vi "Copy of Create calibration array.vi"() -> ()   [LabVIEW 2009, in "Varian Magnet.lvclass"]
uses:
  Varian Magnet.lvclass
panel:
  in  "# of points":dbl
  out "Rate":dbl[unit]
  out "Time":dbl[unit]
  out "Current Field":dbl[](array[numeric])
  in  "Start":bool
  in  "stop":bool
  out "step size":dbl[unit]
  in  "ending field":dbl[unit]
  in  "starting field":dbl[unit]
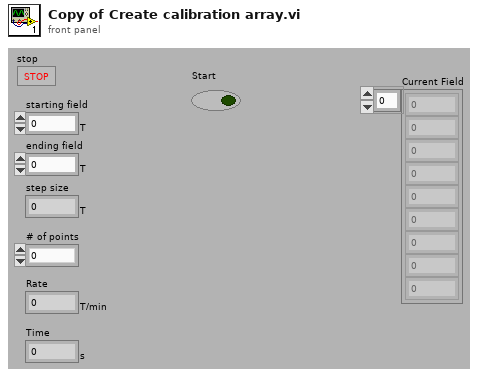
[diagram p1: front panel]
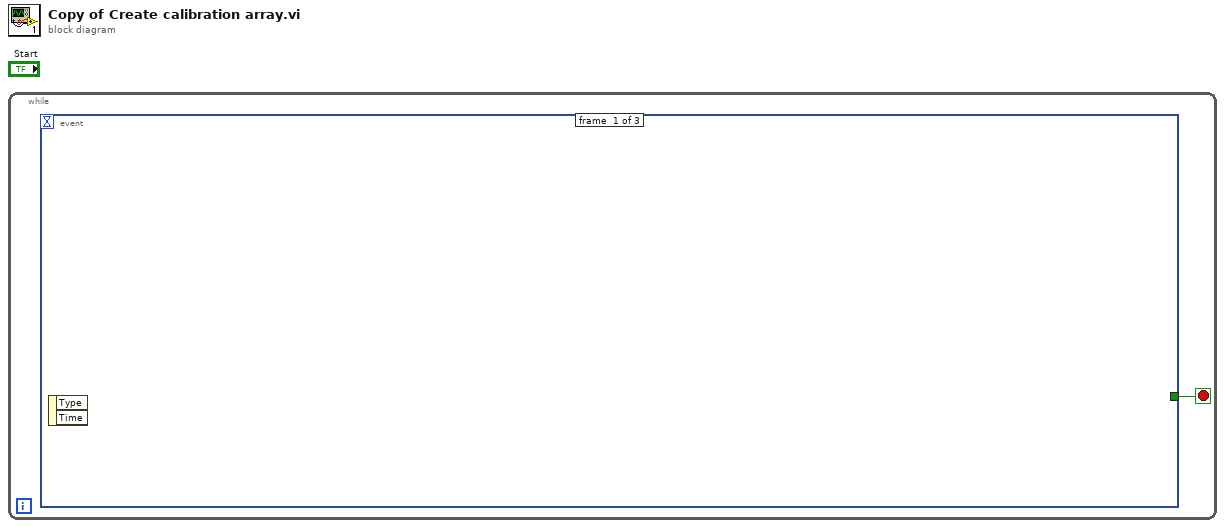
[diagram p0: block diagram]
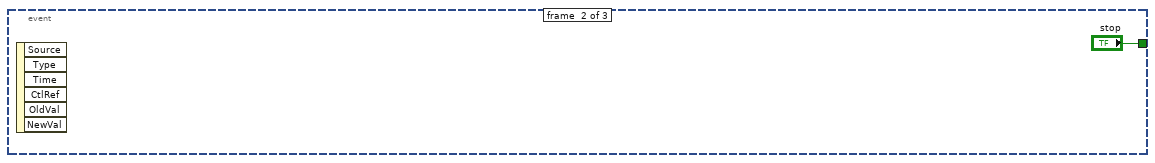
[diagram p2: hidden frame]
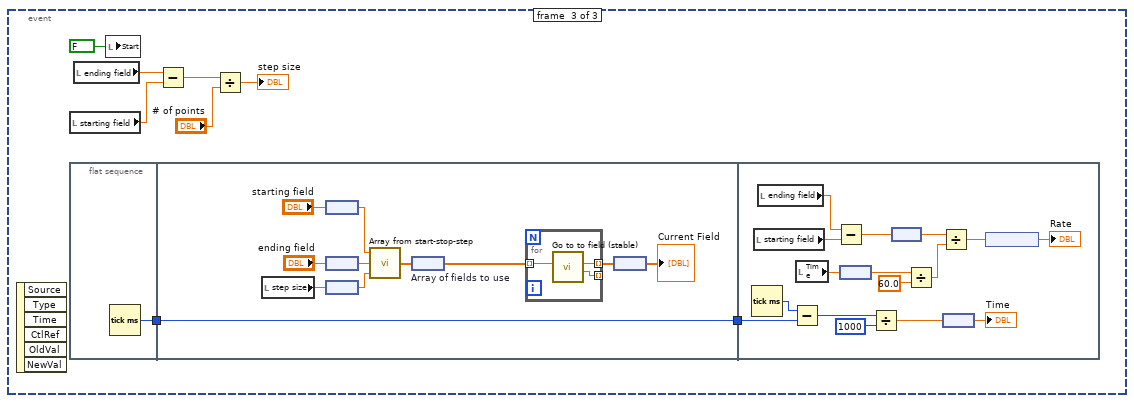
[diagram p3: hidden frame]
diagram:
  n1 = while {
    stop <- w1 stop-if-true
    n2 = event shown="[2] \"Start\": Value Change" {
      selector: _ -> [_ _ _]
      dyn-events: _ -> [_ _ _]
      timeout: _ -> [_ _ _]
      tunnel: [_ "stop" _] -> w1
      event #0 {
        n3 = event-data() -> ()  [unwired: 3 out]
      }
      event #1 {
        n4 = event-data() -> ()  [unwired: 7 out]
      }
      event #2 {
        n5 = event-data() -> ()  [unwired: 7 out]
        n6 = local read "starting field"() -> (w5:dbl[unit])
        n7 = flat-sequence {
          tunnel: [w11] -> w9
          tunnel: w9 -> [w13]
          tunnel: [w13] -> w8
          tunnel: w8 -> [w40]
          frame #0 {
            n8 = Tick Count (ms)() -> (millisecond timer value=w11:u32)
          }
          frame #1 {
            n9 = local read "step size"() -> (w12:dbl[unit])
            n10 = node("starting field") -> (w18:dbl)
            n11 = node("ending field") -> (w20:dbl)
            n12 = node(w12) -> (w17:dbl)
            n13 = call "Array from start-stop-step.vi"("Step"=w17, "Stop"=w20, "Start"=w18) -> ("Array of numbers"=w19:dbl[])
            n14 = node "Array of fields to use"(w19) -> (w16:dbl[unit][])
            n15 = for {
              tunnel: w16 -> [w25] mode=indexing
              tunnel: [w24] -> w15 mode=indexing
              tunnel: [w23] -> _ mode=indexing
              n16 = call "Go to to field (stable).vi"("Desired field"=w25) -> ("Current control voltage"=w23:dbl, "Current field"=w24:dbl[unit])  [unwired: 2 in, 7 out]
            }
            n17 = node(w15) -> (→"Current Field":dbl[])
          }
          frame #2 {
            n18 = Tick Count (ms)() -> (millisecond timer value=w41:u32)
            n19 = local read "starting field"() -> (w37:dbl[unit])
            n20 = local read "ending field"() -> (w36:dbl[unit])
            n21 = Subtract(x=w41, y=w40) -> (x-y=w39:u32)
            n22 = local read "Time"() -> (w31:dbl[unit])
            n23 = Subtract(x=w36, y=w37) -> (x-y=w28:dbl[unit])
            n24 = node(w31) -> (w30:dbl)
            n25 = Divide(x=w39, y=u32 1000) -> (x/y=w33:dbl)
            n26 = node(w28) -> (w27:dbl)
            n27 = Divide(x=w30, y=60.0) -> (x/y=w34:dbl)
            n28 = Divide(x=w27, y=w34) -> (x/y=w29:dbl)
            n29 = node(w33) -> (→"Time":dbl[unit])
            n30 = node(w29) -> (→"Rate":dbl[unit])
          }
        }
        n31 = local read "ending field"() -> (w4:dbl[unit])
        n32 = local write "Start"(FALSE ("Create calibration array")) -> ()
        n33 = Subtract(x=w4, y=w5) -> (x-y=w6:dbl[unit])
        n34 = Divide(x=w6, y="# of points") -> (x/y=→"step size":dbl[unit])
      }
    }
  }
